vi "COD质控流程 (子VI).vi"(10 "CODMn量程切换":enum32{"H", "L", "AUTO"}(ring)=enum."AUTO", 11 "COD":bool) -> (2 "CODMn中断报警":bool, 3 "布尔":bool)   [LabVIEW 2016, in "质控单元.lvlib"]
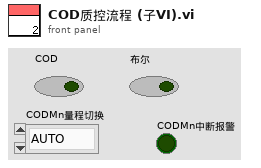
[diagram p1: front panel]
types:
  T1 = enum16{"待机", "启动水样测量", "水样测量中", "启动加标", "启动加标回收", "加标回收测量中", "结束"}
  T2 = cluster{"测量模式":enum16{"水样测量", "标样核查", "零点核查", "跨度核查", "空白测试", "加标回收", "平行样", "校零", "校标"}}
  T3 = cluster{"量程":dbl, "检出限":dbl, "加标前水样浓度":dbl, "加标后水样浓度":dbl, "加标水杯定容体积":dbl, "加标母液浓度":dbl, "加标体积":dbl, "加标回收率":dbl}
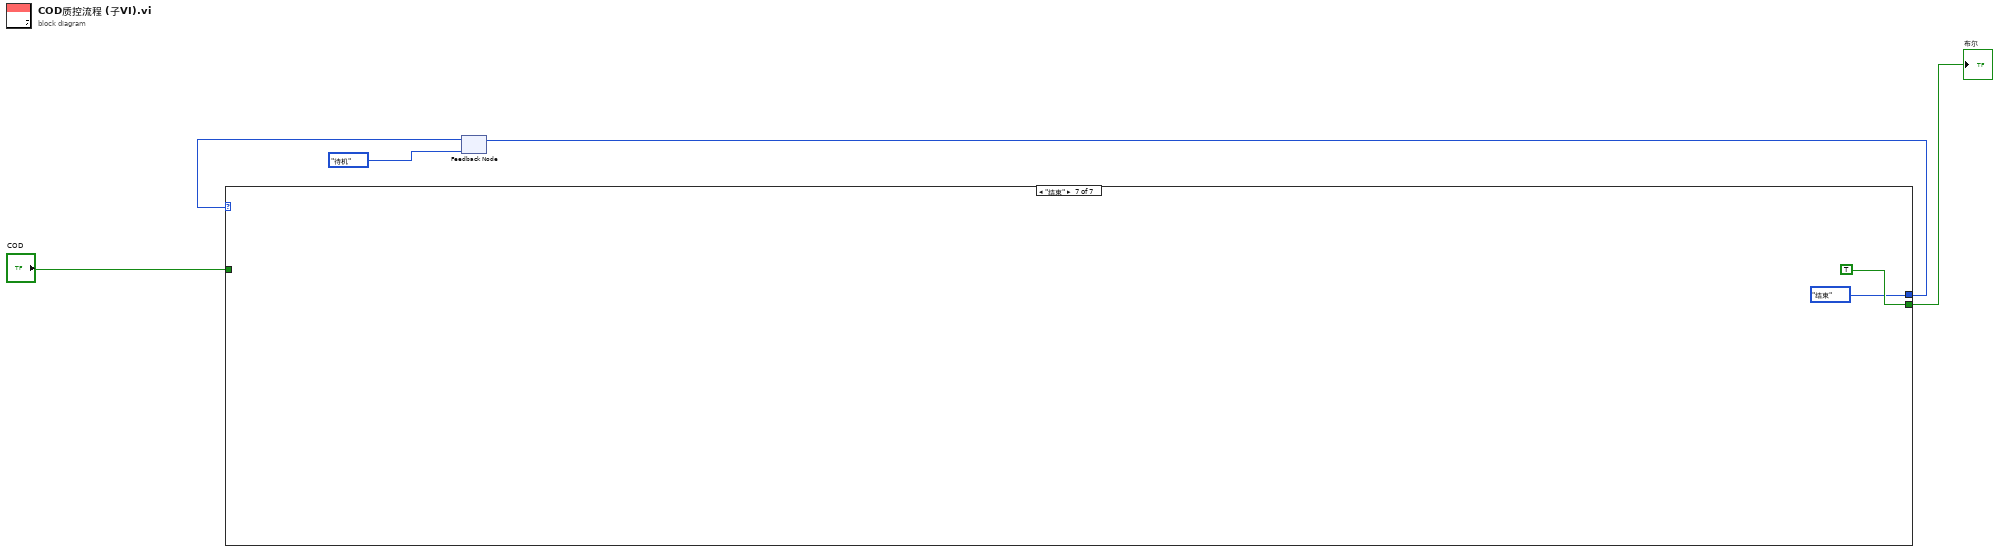
[diagram p0: block diagram]
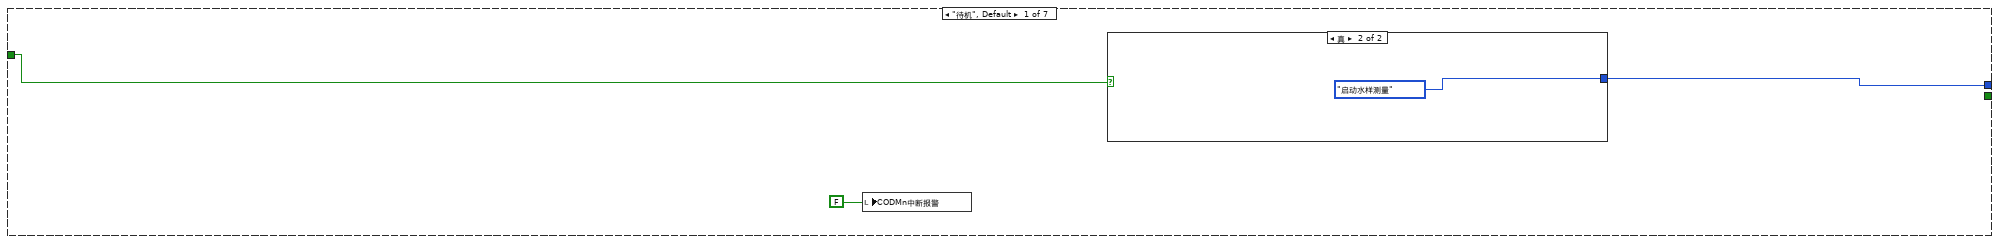
[diagram p2: hidden frame]
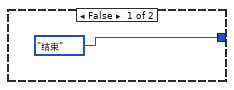
[diagram p3: hidden frame]
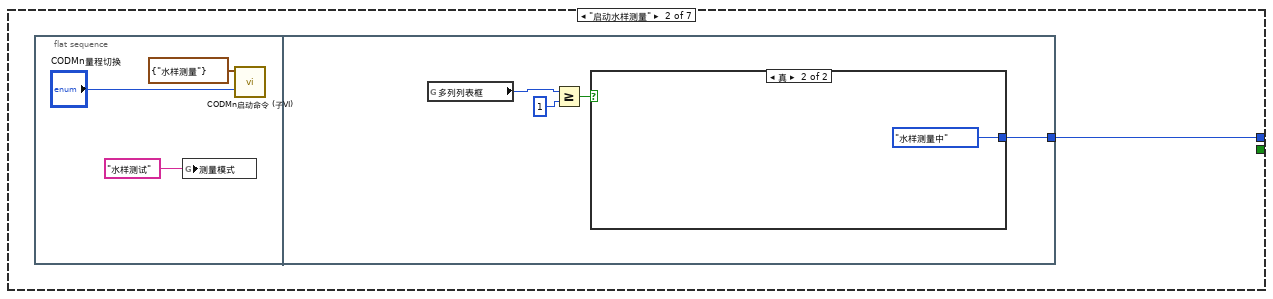
[diagram p4: hidden frame]
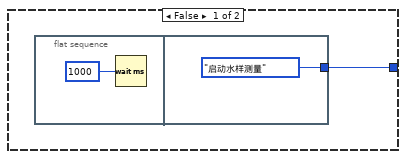
[diagram p5: hidden frame]
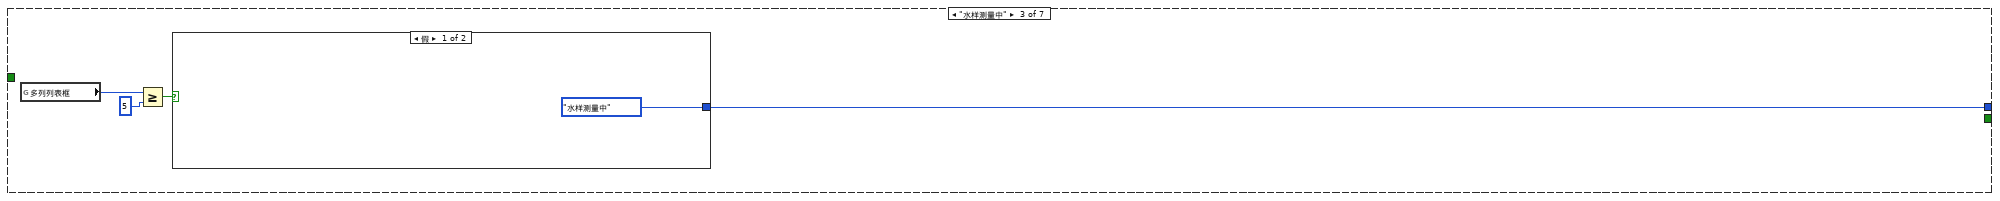
[diagram p6: hidden frame]
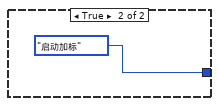
[diagram p7: hidden frame]
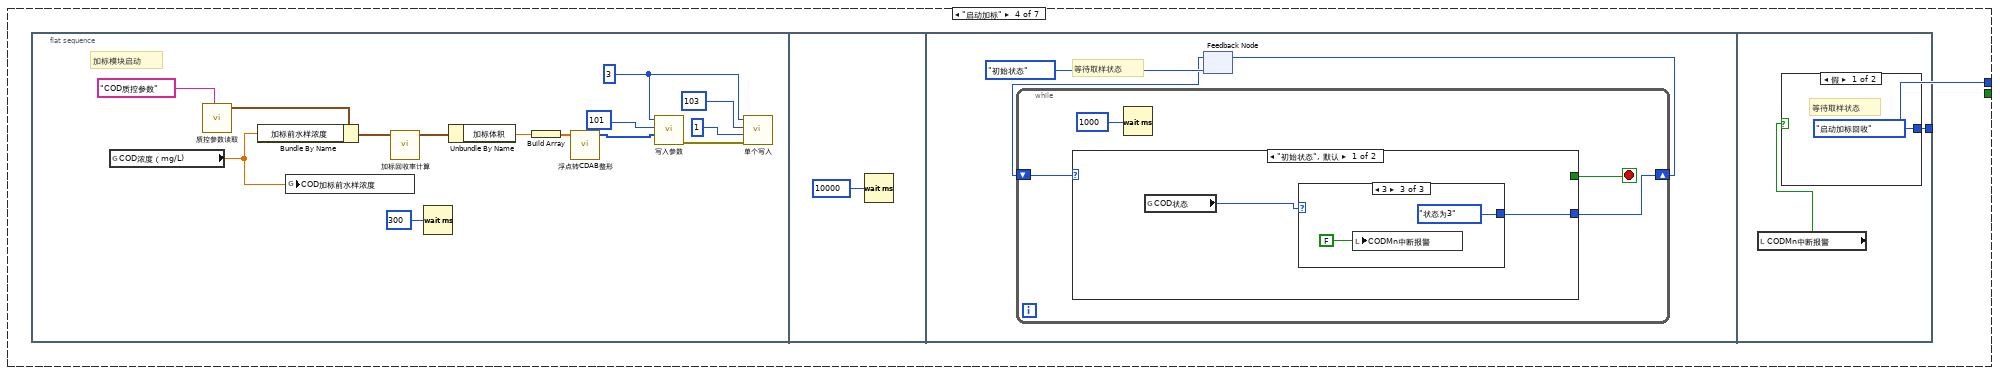
[diagram p8: hidden frame]
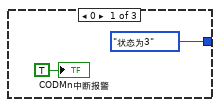
[diagram p9: hidden frame]
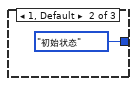
[diagram p10: hidden frame]
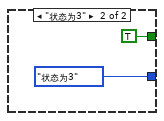
[diagram p11: hidden frame]
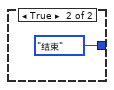
[diagram p12: hidden frame]
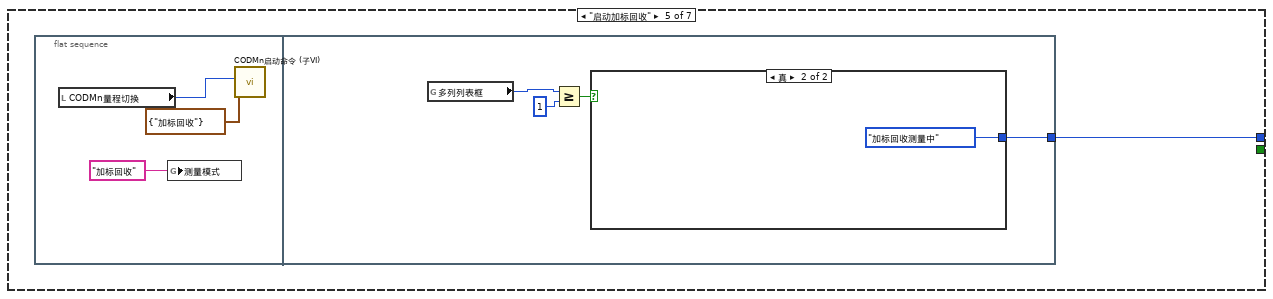
[diagram p13: hidden frame]
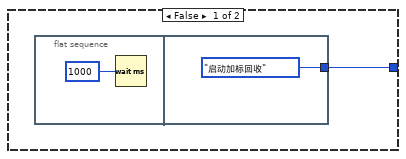
[diagram p14: hidden frame]
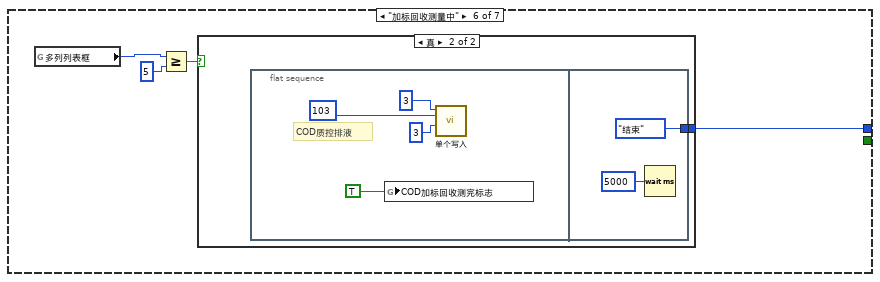
[diagram p15: hidden frame]
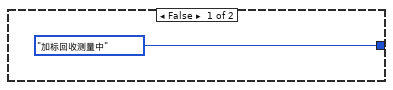
[diagram p16: hidden frame]
diagram:
  n1 = feedback #1(T1."待机") -> (w3:T1)
  n2 = case shown="\"结束\"" w3 {
    tunnel: [w8 w11 w23 w29 w65 w77 T1."结束"] -> w4
    tunnel: [_ _ _ _ _ _ TRUE] -> w2
    tunnel: "COD" -> [w7 _ _ _ _ _ _]
    frame "待机", Default {
      n3 = local write "CODMn中断报警"(FALSE ("CODMn中断报警")) -> ()
      n4 = case shown="真" w7 {
        tunnel: [T1."结束" T1."启动水样测量"] -> w8
        frame False {
        }
        frame True {
        }
      }
    }
    frame "启动水样测量" {
      n5 = flat-sequence {
        tunnel: [w15] -> w11
        frame #0 {
          n6 = global write "COD测量模式全局.vi" "测量模式"("水样测试" ("测量模式")) -> ()
          n7 = call "CODMn启动命令 (子VI).vi"("CODMn量程切换"="CODMn量程切换", "启动测量模式"=T2 {"测量模式"=enum."水样测量"}) -> ()  [unwired: 10 in]
        }
        frame #1 {
          n8 = global read "运行时序全局变量.vi" "多列列表框"() -> (w18:i32)
          n9 = Greater Or Equal?(x=w18, y=1) -> (x >= y?=w17:bool)
          n10 = case shown="真" w17 {
            tunnel: [w19 T1."水样测量中"] -> w15
            frame False {
              n11 = flat-sequence {
                tunnel: [T1."启动水样测量"] -> w19
                frame #0 {
                  n12 = Wait (ms)(milliseconds to wait=u32 1000 ("等待时间（毫秒）")) -> ()  [unwired: 1 out]
                }
                frame #1 {
                }
              }
            }
            frame True {
            }
          }
        }
      }
    }
    frame "水样测量中" {
      n13 = global read "运行时序全局变量.vi" "多列列表框"() -> (w24:i32)
      n14 = Greater Or Equal?(x=w24, y=5) -> (x >= y?=w25:bool)
      n15 = case shown="假" w25 {
        tunnel: [T1."水样测量中" T1."启动加标"] -> w23
        frame False {
        }
        frame True {
        }
      }
    }
    frame "启动加标" {
      n16 = flat-sequence {
        tunnel: [w62] -> w29
        frame #0 {
          w31 = u16 3 ("value")
          # "加标模块启动"
          n17 = global read "COD浓度全局变量.vi" "COD浓度（mg/L)"() -> (w32:dbl)
          n18 = call "质控参数读取.vi"("section"="COD质控参数") -> ("参数"=w41:T3)  [unwired: 9 in, 1 out]
          n19 = Bundle By Name(cluster=w41, "加标前水样浓度"=w32) -> (w42:T3)
          n20 = global write "水样浓度全局.vi" "COD加标前水样浓度"(w32) -> ()
          n21 = call "加标回收率计算.vi"("参数"=w42) -> ("参数 out"=w40:T3)  [unwired: 10 in]
          n22 = Wait (ms)(milliseconds to wait=u32 300 ("等待时间（毫秒）")) -> ()  [unwired: 1 out]
          n23 = Unbundle By Name(w40) -> ("加标体积"=w33:dbl)
          n24 = Build Array(w33) -> (w39:dbl[])
          n25 = call "浮点转CDAB整形.vi"("浮点数"=w39) -> ("CDAB整形输出"=w34:u16[])  [unwired: 10 in]
          n26 = call "写入参数.vi"("values"=w34, "starting address"=u16 101, "Slave ID"=w31) -> ("error out"=w38:errorcluster)  [unwired: 8 in]
          n27 = call "单个写入.vi"("Error in"=w38, "value"=u16 1, "address"=u16 103, "Slave ID"=w31) -> ()  [unwired: 7 in, 1 out]
        }
        frame #1 {
          n28 = Wait (ms)(milliseconds to wait=u32 10000 ("等待时间（毫秒）")) -> ()  [unwired: 1 out]
        }
        frame #2 {
          # "等待取样状态"
          n29 = feedback #2(enum16{"初始状态", "状态为3"}."初始状态") -> (w46:enum16{"初始状态", "状态为3"})
          n30 = while {
            shift-right: [w50] -> w45
            shift-left: w46 -> [w51]
            stop <- w49 stop-if-true
            n31 = case shown="\"初始状态\", 默认" w51 {
              tunnel: [w53 enum16{"初始状态", "状态为3"}."状态为3"] -> w50
              tunnel: [_ TRUE] -> w49
              frame "初始状态", Default {
                n32 = global read "氨氮加标回收状态全局变量.vi" "COD状态"() -> (w52:u16)
                n33 = case shown="3" w52 {
                  tunnel: [enum16{"初始状态", "状态为3"}."状态为3" enum16{"初始状态", "状态为3"}."初始状态" enum16{"初始状态", "状态为3"}."状态为3"] -> w53
                  frame 0 {
                    "CODMn中断报警" <- TRUE ("CODMn中断报警")
                  }
                  frame 1, Default {
                  }
                  frame 3 {
                    n34 = local write "CODMn中断报警"(FALSE ("CODMn中断报警")) -> ()
                  }
                }
              }
              frame "状态为3" {
              }
            }
            n35 = Wait (ms)(milliseconds to wait=u32 1000 ("等待时间（毫秒）")) -> ()  [unwired: 1 out]
          }
          n36 = feedback-in #2(w45) -> ()
        }
        frame #3 {
          n37 = local read "CODMn中断报警"() -> (w61:bool)
          n38 = case shown="假" w61 {
            tunnel: [T1."启动加标回收" T1."结束"] -> w62
            frame False {
              # "等待取样状态"
            }
            frame True {
            }
          }
        }
      }
    }
    frame "启动加标回收" {
      n39 = flat-sequence {
        tunnel: [w69] -> w65
        frame #0 {
          n40 = local read "CODMn量程切换"() -> (w67:enum32{"H", "L", "AUTO"})
          n41 = global write "COD测量模式全局.vi" "测量模式"("加标回收" ("测量模式")) -> ()
          n42 = call "CODMn启动命令 (子VI).vi"("CODMn量程切换"=w67, "启动测量模式"=T2 {"测量模式"=enum."加标回收"}) -> ()  [unwired: 10 in]
        }
        frame #1 {
          n43 = global read "运行时序全局变量.vi" "多列列表框"() -> (w70:i32)
          n44 = Greater Or Equal?(x=w70, y=1) -> (x >= y?=w71:bool)
          n45 = case shown="真" w71 {
            tunnel: [w73 T1."加标回收测量中"] -> w69
            frame False {
              n46 = flat-sequence {
                tunnel: [T1."启动加标回收"] -> w73
                frame #0 {
                  n47 = Wait (ms)(milliseconds to wait=u32 1000 ("等待时间（毫秒）")) -> ()  [unwired: 1 out]
                }
                frame #1 {
                }
              }
            }
            frame True {
            }
          }
        }
      }
    }
    frame "加标回收测量中" {
      n48 = global read "运行时序全局变量.vi" "多列列表框"() -> (w78:i32)
      n49 = Greater Or Equal?(x=w78, y=5) -> (x >= y?=w79:bool)
      n50 = case shown="真" w79 {
        tunnel: [T1."加标回收测量中" w82] -> w77
        frame False {
        }
        frame True {
          n51 = flat-sequence {
            tunnel: [T1."结束"] -> w82
            frame #0 {
              # "COD质控排液"
              n52 = global write "质控测完标志全局 1.vi" "COD加标回收测完标志"(TRUE ("COD加标回收测完标志")) -> ()
              n53 = call "单个写入.vi"("value"=u16 3, "address"=u16 103, "Slave ID"=u8 3) -> ()  [unwired: 8 in, 1 out]
            }
            frame #1 {
              n54 = Wait (ms)(milliseconds to wait=u32 5000 ("等待时间（毫秒）")) -> ()  [unwired: 1 out]
            }
          }
        }
      }
    }
    frame "结束" {
    }
  }
  "布尔" <- w2
  n55 = feedback-in #1(w4) -> ()
